vi "MX Initial.vi"(8 "错误输入":errorcluster) -> (0 "错误输出":errorcluster, 3 "引用输出":refnum<k7>)   [LabVIEW 2017]
panel:
  out "Open":i32
  in  "ActUtlTypeLib.IActUtlType":refnum<k7>
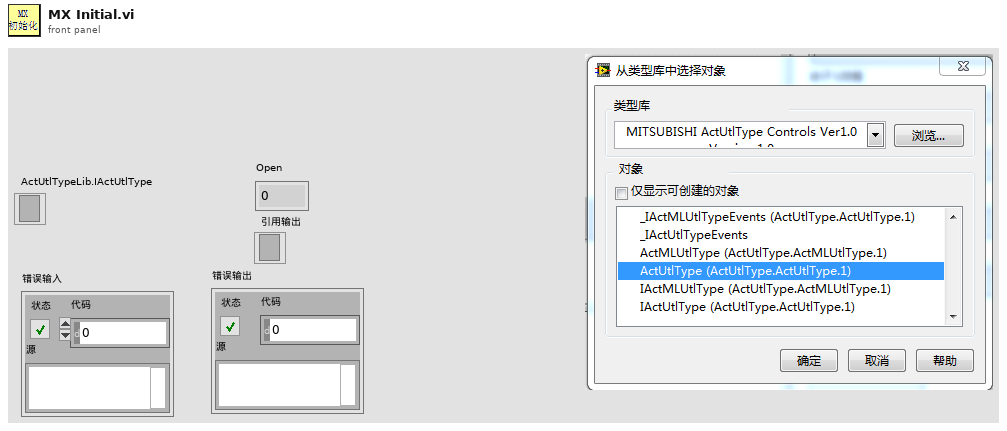
[diagram p1: front panel]
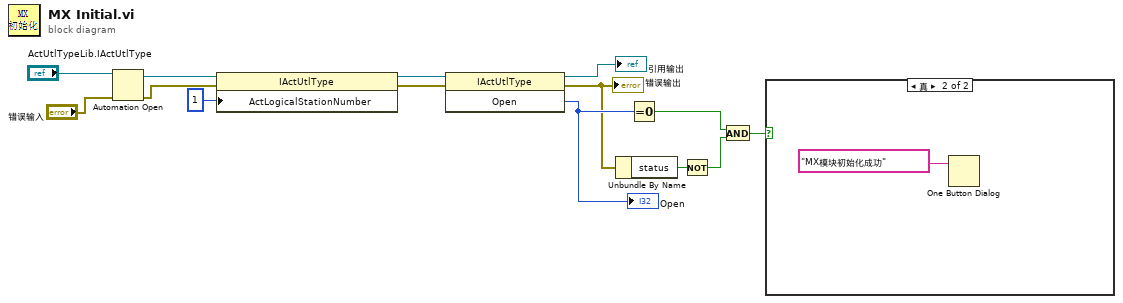
[diagram p0: block diagram]
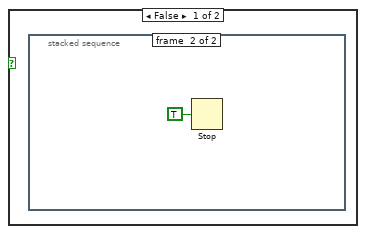
[diagram p2: hidden frame]
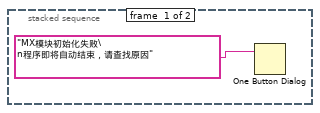
[diagram p3: hidden frame]
diagram:
  n1 = Automation Open(error in (no error)="错误输入", Automation Refnum="ActUtlTypeLib.IActUtlType") -> (Automation Refnum=w12:refnum<k7>, error out=w11:errorcluster)  [unwired: 2 in]
  n2 = property on="属性节点" class="IActUtlType"(reference=w12, error in=w11, "ActLogicalStationNumber"=1) -> (reference out=w9:refnum<k7>, error out=w8:errorcluster)
  n3 = invoke on="调用节点" class="IActUtlType" method="Open"(reference=w9, error in=w8) -> (reference out=→"引用输出":refnum<k7>, error out=w6:errorcluster, "Open"=w7:i32)  [unwired: 1 in]
  "Open" <- w7
  "错误输出" <- w6
  n4 = Unbundle By Name(w6) -> ("status"=w5:bool)
  n5 = Equal To 0?(x=w7) -> (x = 0?=w4:bool)
  n6 = Not(x=w5) -> (.not. x?=w3:bool)
  n7 = And(x=w4, y=w3) -> (x .and. y?=w2:bool)
  n8 = case shown="真" w2 {
    frame False {
      n9 = stacked-sequence {
        frame #0 {
          n10 = One Button Dialog(message="MX模块初始化失败\n程序即将自动结束，请查找原因" ("消息")) -> ()  [unwired: 1 in, 1 out]
        }
        frame #1 {
          n11 = Stop(stop? (T)=TRUE ("停止？(T)")) -> ()
        }
      }
    }
    frame True {
      n12 = One Button Dialog(message="MX模块初始化成功" ("消息")) -> ()  [unwired: 1 in, 1 out]
    }
  }
